vi "variable PID.vi"(2 "PID output":dbl, 3 "Motor single.lvclass":refnum<class "Motor single.lvclass">) -> (0 "PID":cluster{"Kp":dbl, "Ki":dbl, "Kd":dbl})   [LabVIEW 2019, in "Motor single.lvclass"]
uses:
  Motor single.lvclass
  Motor single.lvclass/Motor single.ctl
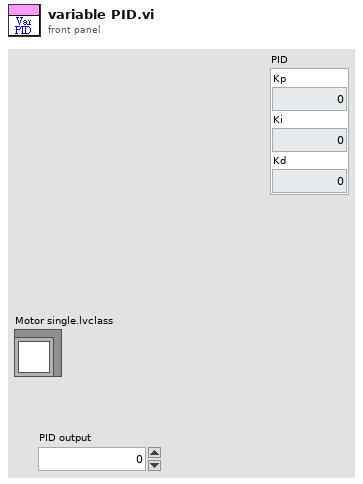
[diagram p1: front panel]
types:
  T1 = typedef "Motor single.lvclass/Variable PID(Kp).ctl" = cluster{"Enable variable PID(Kp)":bool, "Variable PID(Kp)range":dbl, "Variable MODE":T2}
  T2 = typedef "Motor single.lvclass/Variable PID(Kp) mode enum.ctl" = enum16{"Log", "Sin&Cos", "Linear", "reverse Log", "const"}
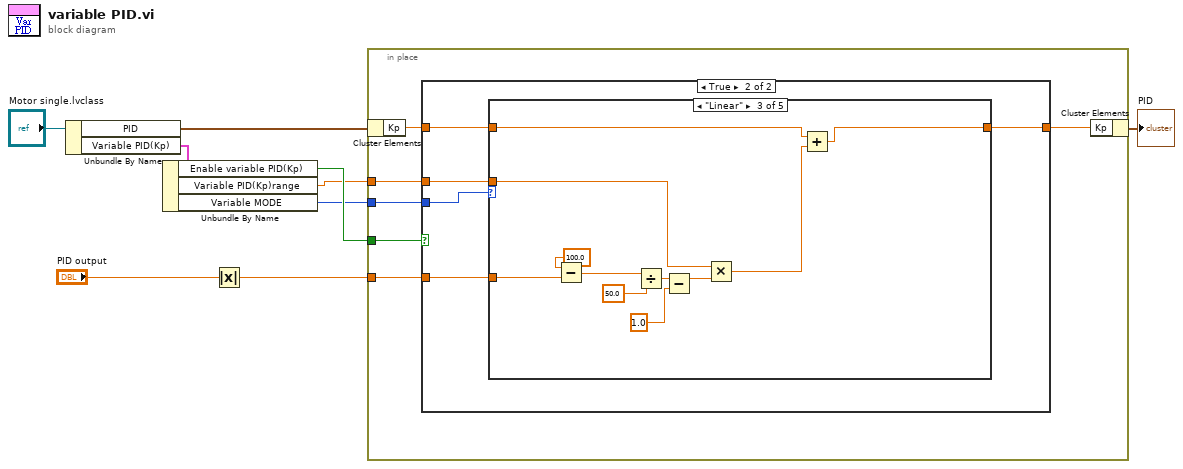
[diagram p0: block diagram]
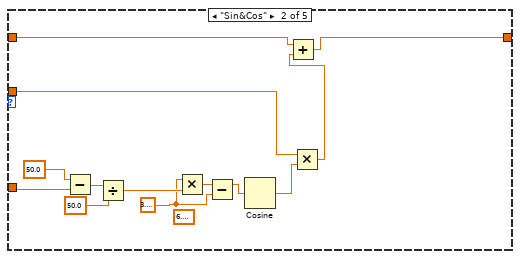
[diagram p4: hidden frame]
diagram:
  n1 = Unbundle By Name("Motor single.lvclass") -> ("PID"=w8:cluster{"Kp":dbl, "Ki":dbl, "Kd":dbl}, "Variable PID(Kp)"=w7:T1)
  n2 = Unbundle By Name(w7) -> ("Enable variable PID(Kp)"=w6:bool, "Variable PID(Kp)range"=w3:dbl, "Variable MODE"=w5:T2)
  n3 = Absolute Value(x="PID output") -> (abs(x)=w1:dbl)
  n4 = in-place {
    in-place-border: w6 -> [w15]
    in-place-border: w5 -> [w12]
    in-place-border: w1 -> [w11]
    in-place-border: w3 -> [w10]
    n5 = in-place-cluster #1(w8) -> ("Kp"=w14:dbl)
    n6 = case shown="True" w15 {
      tunnel: w14 -> [w16 w19]
      tunnel: [w16 w20] -> w13
      tunnel: w12 -> [_ w21]
      tunnel: w11 -> [_ w18]
      tunnel: w10 -> [_ w17]
      frame False {
      }
      frame True {
        n7 = case shown="\"Linear\"" w21 {
          tunnel: [w22 w30 w36 w47 w48] -> w20
          tunnel: w19 -> [w22 w31 w38 w47 w48]
          tunnel: w18 -> [_ w34 w43 _ _]
          tunnel: w17 -> [_ w29 w41 _ _]
          frame "Log", Default {
          }
          frame "Sin&Cos" {
            (unwired) 6.283185307179586
            w23 = 3.141592653589793
            n8 = Subtract(x=50.0, y=w34) -> (x-y=w32:dbl)
            n9 = Divide(x=w32, y=50.0) -> (x/y=w26:dbl)
            n10 = Multiply(x=w23, y=w26) -> (x*y=w25:dbl)
            n11 = Subtract(x=w25, y=w23) -> (x-y=w24:dbl)
            n12 = Cosine(x=w24) -> (cos(x)=w28:dbl)
            n13 = Multiply(x=w29, y=w28) -> (x*y=w27:dbl)
            n14 = Add(x=w31, y=w27) -> (x+y=w30:dbl)
          }
          frame "Linear" {
            n15 = Subtract(x=100.0, y=w43) -> (x-y=w44:dbl)
            n16 = Divide(x=w44, y=50.0) -> (x/y=w42:dbl)
            n17 = Subtract(x=w42, y=1.0) -> (x-y=w40:dbl)
            n18 = Multiply(x=w41, y=w40) -> (x*y=w37:dbl)
            n19 = Add(x=w38, y=w37) -> (x+y=w36:dbl)
          }
          frame "reverse Log" {
          }
          frame "const" {
          }
        }
      }
    }
    n20 = in-place-cluster #1("Kp"=w13) -> (→"PID":cluster{"Kp":dbl, "Ki":dbl, "Kd":dbl})
  }
